vi "PIDController_Pack_InputLimits.vi"(9 "Continuous":bool, 10 "MinInput":dbl, 11 "MaxInput":dbl) -> (3 "PID Input Limits":T1)   [LabVIEW 2019, in "Trajectory_Library.lvlib"]
doc: "Convience function to pack individual input limit values into a cluster to pass to the PID controller\n\nInputs:\n\n - Max Input -- The maximum allowed input The units are the same as the Setpoint (SP) and Process variable (PV)\n - Min Input -- The minimum allowed input value The units are the same as the Setpoint (SP) and Process variable (PV)\n - Continuous -- Boolean indicating that the inputs wrap from the maximum value to the miimum value.. (Example - gyro and heading control)\n\nOutput:\n - PID Input Limits -- Cluster containing the input values"
uses:
  Trajectory_Library.lvlib
  TypeDef/PID_INPUT_LIMITS.ctl
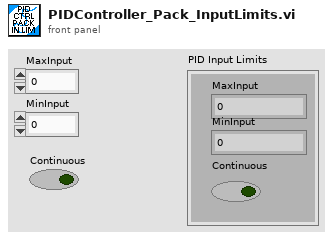
[diagram p1: front panel]
types:
  T1 = typedef "Trajectory_Library.lvlib/PID_INPUT_LIMITS.ctl" = cluster{"MaxInput":dbl, "MinInput":dbl, "Continuous":bool}
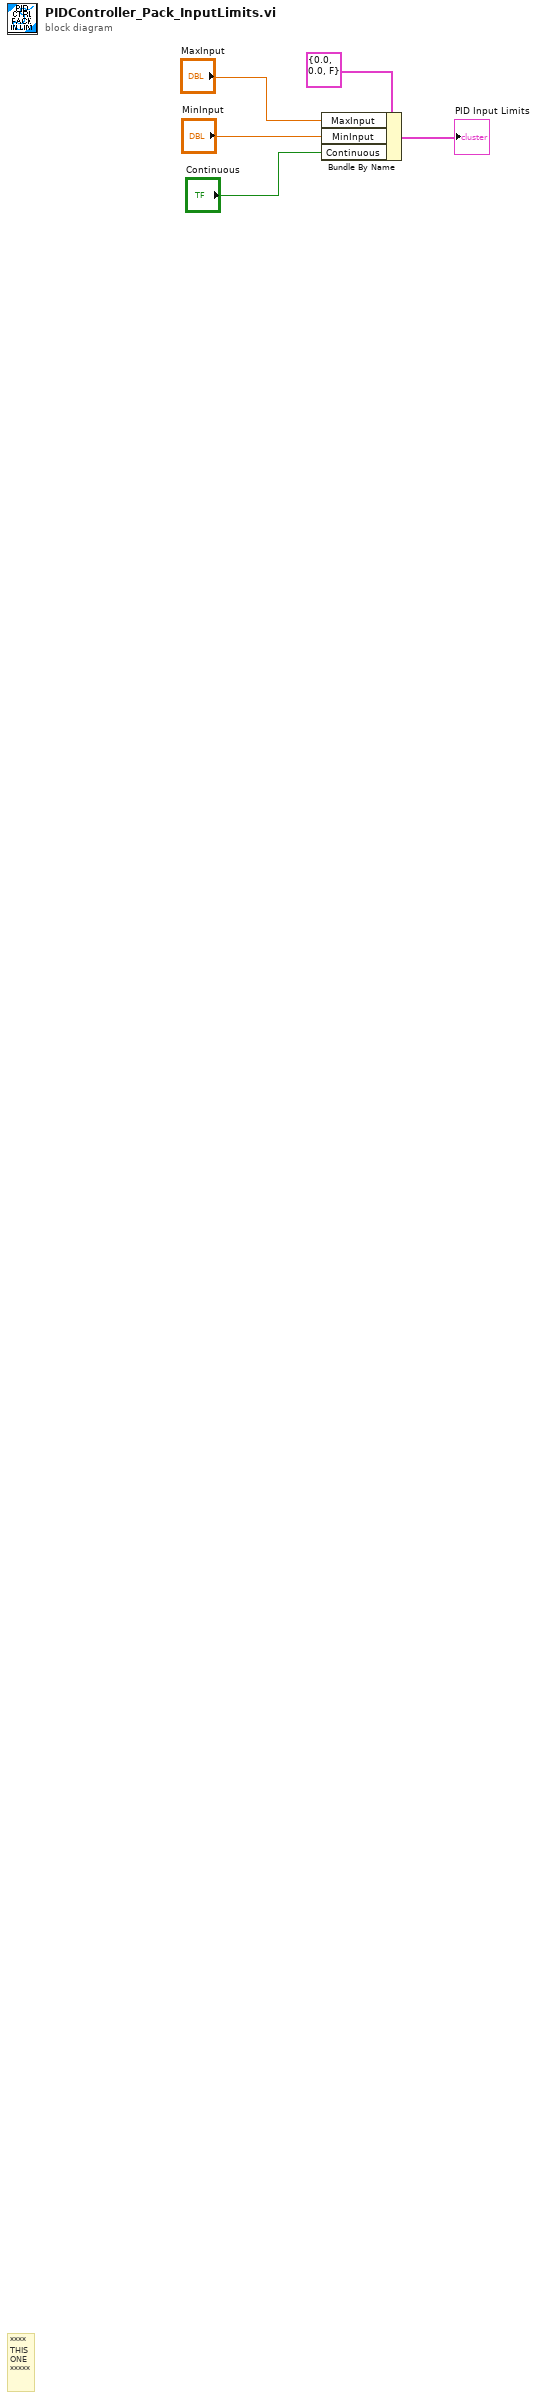
[diagram p0: block diagram]
diagram:
  # "****\nTHIS\nONE\n*****"
  n1 = Bundle By Name(cluster=T1 {"MaxInput"=0.0, "MinInput"=0.0, "Continuous"=FALSE} ("PID Input Limits"), "MaxInput"="MaxInput", "MinInput"="MinInput", "Continuous"="Continuous") -> (→"PID Input Limits":T1)
